vi "S8300E_RTC_Compare_Default.vi"() -> ()   [LabVIEW 2011]
uses:
  Instance           4 29Saved   Mojo_RTC_SFCS_Compare .vi
panel:
  out "Tolerance sec":string
  out "UUT sec":i32
  out "UUT min":i32
  out "UUT hour":i32
  out "UUT Day":i32
  out "UUT  Month":i32
  out "UUT Year":i32
  out "UUT-DateTime":string
  out "VISA resource name out":refnum<visa-resource-name>
  out "Start Time":u32
  out "RTC Elapsed Time":dbl
  out "TimeGap(sec)":dbl format="%#_8f"
  out "sec":i32
  out "minute":i32
  out "hour":i32
  out "day":i32
  out "month":i32
  out "year":i32
  # "Error Code:RTC\nError Code:UART"
  # "網路時間與S8300E 時間比較\nDefault Time compare to S8300E RTC Time"
  # "2015-6-12"
  # "COM9, Baud 115200"
  # "Default  Time:"
  # "UUT-Date-Time:"
  # "Default Time:2011/1/1 00:00:00"
  # "Formula :TimeGap=UUT Time -Default Time"
  # ">"
  # "Pass Criteria"
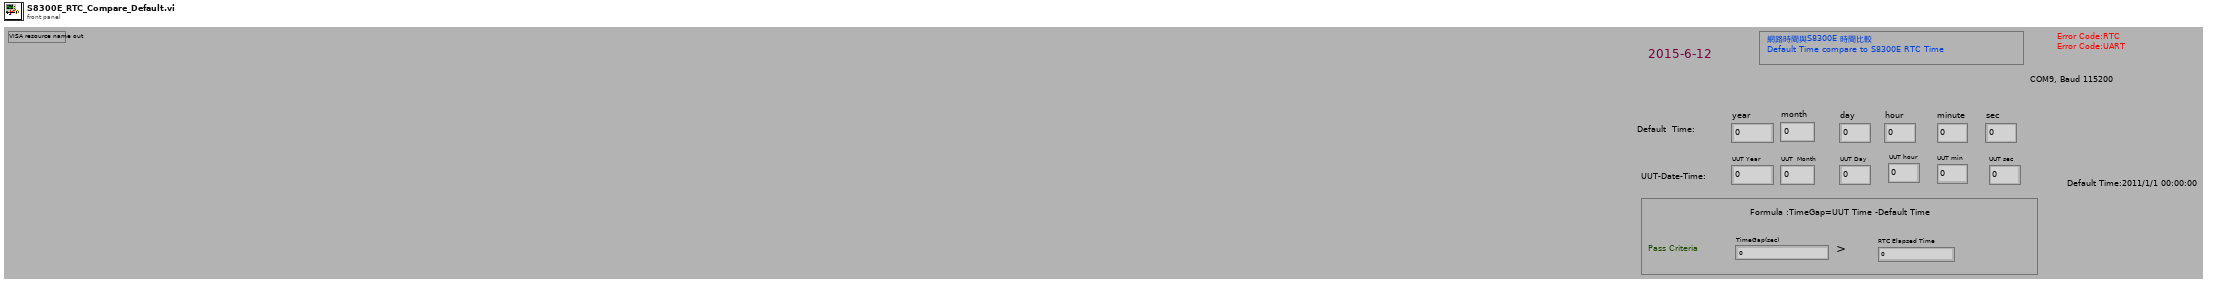
[diagram p1: front panel]
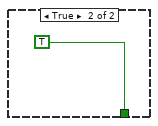
[diagram p5: hidden frame]
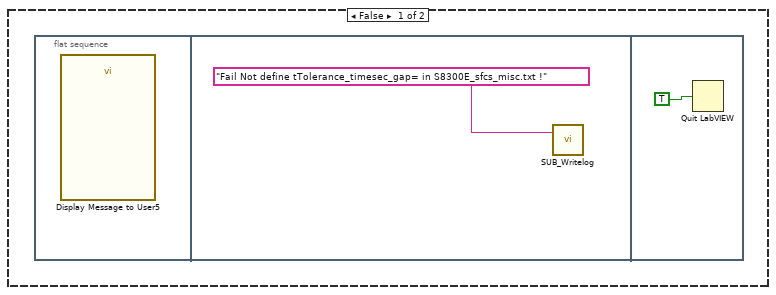
[diagram p6: hidden frame]
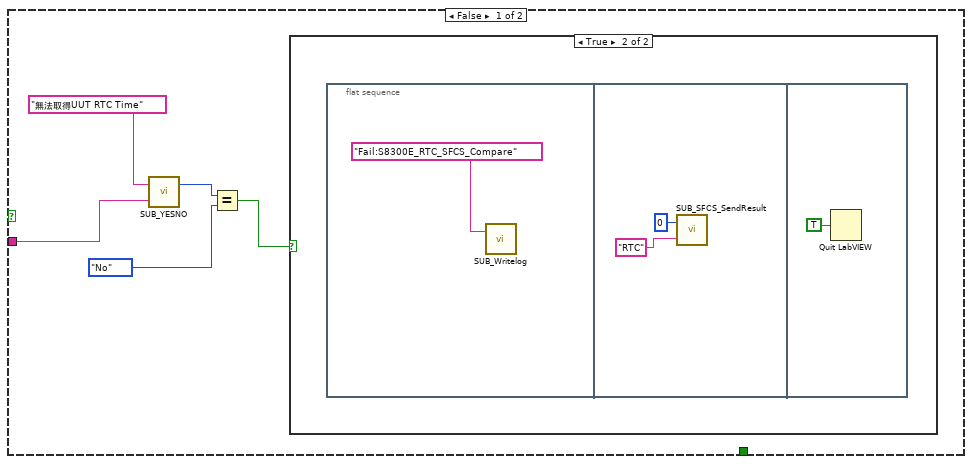
[diagram p8: hidden frame]
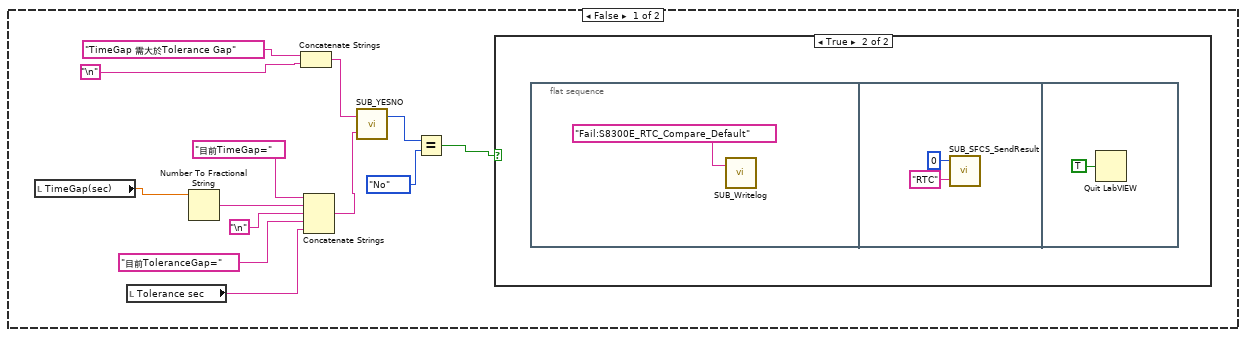
[diagram p10: hidden frame]
diagram:
  n1 = flat-sequence {
    frame #0 {
      n2 = Tick Count (ms)() -> (millisecond timer value=→"Start Time":u32)
    }
    frame #1 {
      n3 = call "SUB_COM1_CLOSE.vi"("VISA resource name"=refnum<visa-resource-name> "COM9") -> ()  [unwired: 3 in]
    }
    frame #2 {
      n4 = case shown="True" TRUE {
        frame False {
        }
        frame True {
          n5 = call "SUB_COM9_INIT.vi"("baud rate"=u32 115200) -> ("VISA resource name out"=w7:refnum<visa-resource-name>)  [unwired: 1 in, 1 out]
          "VISA resource name out" <- w7
          n6 = call "SUB_COM1Wrt.vi"("VISA resource name"=w7, "write buffer"="\r") -> ("duplicate VISA resource name"=w4:refnum<visa-resource-name>)  [unwired: 1 in, 1 out]
          n7 = call "SUB_ContinueCom1Read.vi"("Numeric"=1200, "duplicate VISA resource name 2"=w4) -> ()  [unwired: 1 in, 3 out]
        }
      }
    }
    frame #3 {
      n8 = case shown="True" TRUE {
        frame False {
        }
        frame True {
          n9 = while {
            stop <- w19 stop-if-true
            w10 = "\r"
            n10 = local read "VISA resource name out"() -> (w18:refnum<visa-resource-name>)
            n11 = Concatenate Strings(w10, w10, w10) -> (w11:string)
            n12 = call "SUB_COM1Wrt.vi"("VISA resource name"=w18, "write buffer"=w11) -> ("duplicate VISA resource name"=w14:refnum<visa-resource-name>)  [unwired: 1 in, 1 out]
            n13 = Tick Count (ms)() -> (millisecond timer value=w13:u32)
            n14 = call "SUB_READ_COM1_FindString_timeout.vi"("Find this String"="S8300E", "Timeout Seccond"=3.0, "Begin time"=w13, "duplicate VISA resource name 2"=w14) -> ("Output String"=w16:string, "Found String"=w15:bool)  [unwired: 1 in, 1 out]
            n15 = case shown="False" w15 {
              tunnel: w16 -> [w24 _]
              tunnel: [w20 TRUE] -> w19
              frame False {
                n16 = call "SUB_YESNO.vi"("Debug View"=w24, "Status"="UART無正確反應!需有S8300E字串") -> ("yes/no"=w23:enum32{"No Selection", "Yes", "No", "None"})  [unwired: 1 in]
                n17 = Equal?(x=w23, y=enum32{"No Selection", "Yes", "No", "None"}."No") -> (x = y?=w21:bool)
                n18 = case shown="True" w21 {
                  tunnel: [_ w26] -> w20
                  frame False {
                  }
                  frame True {
                    n19 = flat-sequence {
                      tunnel: [w30] -> w26
                      frame #0 {
                        n20 = call "SUB_Writelog.vi"("Pass/Fail"="Fail:S8300E_RTC_SFCS_Compare") -> ()  [unwired: 2 in]
                      }
                      frame #1 {
                        n21 = call "SUB_SFCS_SendResult.vi"("ErrorCode"="UART", "PASS_Fail (1/0)"=i8 0) -> ()  [unwired: 1 out]
                      }
                      frame #2 {
                        w30 = TRUE ("quit? (T)")
                        n22 = Quit LabVIEW(quit? (T)=w30) -> ()
                      }
                    }
                  }
                }
              }
              frame True {
              }
            }
          }
        }
      }
    }
    frame #4 {
      n23 = call "SUB_Read_specifFile.vi"("name or relative path"="S8300E_sfcs_misc.txt") -> ("text"=w33:string)  [unwired: 1 in, 1 out]
      n24 = call "SUB_FindSpecificString.vi"("Find this String"="RTC_DEFAULT_ELAPSED_TIME=", "String data"=w33) -> ("before \"; \" string"=w34:string, "Found"=w35:bool)  [unwired: 2 in]
      n25 = case shown="True" w35 {
        tunnel: w34 -> [_ w40]
        frame False {
          n26 = flat-sequence {
            frame #0 {
              n27 = call "Display Message to User5"() -> ()  [unwired: 10 in, 2 out]
            }
            frame #1 {
              n28 = call "SUB_Writelog.vi"("Pass/Fail"="Fail Not define tTolerance_timesec_gap= in S8300E_sfcs_misc.txt !") -> ()  [unwired: 2 in]
            }
            frame #2 {
              n29 = Quit LabVIEW(quit? (T)=TRUE) -> ()
            }
          }
        }
        frame True {
          n30 = Fract/Exp String To Number(string=w40) -> (number=→"RTC Elapsed Time":dbl)  [unwired: 3 in, 1 out]
          "Tolerance sec" <- w40
        }
      }
    }
    frame #5 {
      n31 = case shown="True" TRUE {
        frame False {
        }
        frame True {
          n32 = while {
            stop <- w47 stop-if-true
            n33 = Concatenate Strings("./rtc.sh -r" ("string"), "\r") -> (w53:string)
            n34 = Tick Count (ms)() -> (millisecond timer value=w43:u32)
            n35 = local read "VISA resource name out"() -> (w51:refnum<visa-resource-name>)
            n36 = call "SUB_COM1Wrt.vi"("VISA resource name"=w51, "write buffer"=w53) -> ("duplicate VISA resource name"=w44:refnum<visa-resource-name>)  [unwired: 1 in, 1 out]
            n37 = call "SUB_READ_COM1_FindString_timeout.vi"("Find this String"="PASSED=", "Timeout Seccond"=3.0, "Begin time"=w43, "duplicate VISA resource name 2"=w44) -> ("Output String"=w46:string)  [unwired: 1 in, 2 out]
            n38 = call "SUB_FindSpecificString.vi"("Find this String"="PASSED=", "String data"=w46) -> ("before \"; \" string"=→"UUT-DateTime":string, "Found"=w48:bool)  [unwired: 2 in]
            n39 = case shown="True" w48 {
              tunnel: w46 -> [w58 _]
              tunnel: [_ TRUE] -> w47
              frame False {
                n40 = call "SUB_YESNO.vi"("Debug View"=w58, "Status"="無法取得UUT RTC Time") -> ("yes/no"=w57:enum32{"No Selection", "Yes", "No", "None"})  [unwired: 1 in]
                n41 = Equal?(x=w57, y=enum32{"No Selection", "Yes", "No", "None"}."No") -> (x = y?=w55:bool)
                n42 = case shown="True" w55 {
                  frame False {
                  }
                  frame True {
                    n43 = flat-sequence {
                      frame #0 {
                        n44 = call "SUB_Writelog.vi"("Pass/Fail"="Fail:S8300E_RTC_SFCS_Compare") -> ()  [unwired: 2 in]
                      }
                      frame #1 {
                        n45 = call "SUB_SFCS_SendResult.vi"("ErrorCode"="RTC", "PASS_Fail (1/0)"=i8 0) -> ()  [unwired: 1 out]
                      }
                      frame #2 {
                        n46 = Quit LabVIEW(quit? (T)=TRUE) -> ()
                      }
                    }
                  }
                }
              }
              frame True {
              }
            }
          }
        }
      }
    }
    frame #6 {
      n47 = local read "UUT-DateTime"() -> (w71:string)
      n48 = call "SUB_UUT_DatTime_Display.vi"("UUT_DateTime_input"=w71) -> ("UUT sec"=→"UUT sec":i32, "UUT min"=→"UUT min":i32, "UUT hour"=→"UUT hour":i32, "UUT Day"=→"UUT Day":i32, "UUT  Month"=→"UUT  Month":i32, "UUT Year"=→"UUT Year":i32)
    }
    frame #7 {
    }
    frame #8 {
      n49 = while {
        stop <- w82 stop-if-true
        n50 = flat-sequence {
          tunnel: [w85] -> w79
          tunnel: [w84] -> w77
          tunnel: [w83] -> w75
          tunnel: [w91] -> w80
          tunnel: w79 -> [w91]
          tunnel: [w90] -> w78
          tunnel: w77 -> [w90]
          tunnel: [w89] -> w76
          tunnel: w75 -> [w89]
          tunnel: [w88] -> w74
          tunnel: [w87] -> w73
          tunnel: [w86] -> w72
          tunnel: [w99] -> w81
          tunnel: w80 -> [w97]
          tunnel: w78 -> [w96]
          tunnel: w76 -> [w95]
          tunnel: w74 -> [w94]
          tunnel: w73 -> [w93]
          tunnel: w72 -> [w92]
          tunnel: w81 -> [w103]
          tunnel: [w100] -> w82
          frame #0 {
            w83 = 1 ("day")
            w84 = 1 ("month")
            w85 = 2011 ("year")
            "year" <- w85
            "month" <- w84
            "day" <- w83
          }
          frame #1 {
            w88 = 0 ("sec")
            w86 = 0 ("minute")
            w87 = 0 ("hour")
            "hour" <- w87
            "minute" <- w86
            "sec" <- w88
          }
          frame #2 {
            n51 = local read "UUT-DateTime"() -> (w98:string)
            n52 = call "SUB_TimeGAP_SFCS_RTC.vi"("SFCS year"=w97, "UUT_DateTime_input"=w98, "SFCS month"=w96, "SFCS day"=w95, "SFCS hour"=w93, "SFCS minute"=w92, "SFCS second"=w94) -> ("TimeGap(sec)"=w99:dbl)
            "TimeGap(sec)" <- w99
          }
          frame #3 {
            n53 = local read "RTC Elapsed Time"() -> (w102:dbl)
            n54 = Greater?(x=w103, y=w102) -> (0:w101:bool)
            n55 = case shown="True" w101 {
              tunnel: [_ TRUE] -> w100
              frame False {
                n56 = local read "TimeGap(sec)"() -> (w113:dbl)
                n57 = local read "Tolerance sec"() -> (w108:string)
                n58 = Number To Fractional String(number=w113) -> (F-format string=w111:string)  [unwired: 3 in]
                n59 = Concatenate Strings("TimeGap 需大於Tolerance Gap", "\n") -> (w114:string)
                n60 = Concatenate Strings("目前TimeGap=" ("string"), w111, "\n", "目前ToleranceGap=" ("string"), w108) -> (w107:string)
                n61 = call "SUB_YESNO.vi"("Debug View"=w107, "Status"=w114) -> ("yes/no"=w106:enum32{"No Selection", "Yes", "No", "None"})  [unwired: 1 in]
                n62 = Equal?(x=w106, y=enum32{"No Selection", "Yes", "No", "None"}."No") -> (x = y?=w104:bool)
                n63 = case shown="True" w104 {
                  frame False {
                  }
                  frame True {
                    n64 = flat-sequence {
                      frame #0 {
                        n65 = call "SUB_Writelog.vi"("Pass/Fail"="Fail:S8300E_RTC_Compare_Default") -> ()  [unwired: 2 in]
                      }
                      frame #1 {
                        n66 = call "SUB_SFCS_SendResult.vi"("ErrorCode"="RTC", "PASS_Fail (1/0)"=i8 0) -> ()  [unwired: 1 out]
                      }
                      frame #2 {
                        n67 = Quit LabVIEW(quit? (T)=TRUE) -> ()
                      }
                    }
                  }
                }
              }
              frame True {
              }
            }
          }
        }
      }
    }
    frame #9 {
      n68 = call "SUB_COM1_CLOSE.vi"("VISA resource name"=refnum<visa-resource-name> "COM9") -> ()  [unwired: 3 in]
    }
    frame #10 {
      w125 = "\r"
      n69 = local read "TimeGap(sec)"() -> (w127:dbl)
      n70 = local read "UUT-DateTime"() -> (w129:string)
      n71 = Tick Count (ms)() -> (millisecond timer value=w134:u32)
      n72 = local read "Start Time"() -> (w133:u32)
      n73 = call "SUB_CAL_TESTTIME.vi"("Test Item name"="S8300E_RTC_Compare_Default", "Stop tick time"=w134, "Start tick time"=w133) -> ("Test Time output"=w124:string)  [unwired: 2 in]
      n74 = Number To Fractional String(number=w127) -> (F-format string=w126:string)  [unwired: 3 in]
      n75 = Concatenate Strings("Pass :S8300E_RTC_Compare_Default" ("Pass/Fail"), w125, "NO Battery  default Date-Time:", "2011/1/1/00:00:00", w125, "Message From UUT:", w129, w125, "TimeGap=", w126, w125, w124) -> (w136:string)
      n76 = call "SUB_Writelog.vi"("Pass/Fail"=w136) -> ()  [unwired: 2 in]
    }
    frame #11 {
      n77 = Request Deallocation(TRUE ("flag")) -> ()
    }
    frame #12 {
      n78 = Quit LabVIEW(quit? (T)=TRUE) -> ()
    }
  }
